vi "Blowout.vi"(10 "Blowout (ms)":u32=1500, 11 "Delay (ms)":u32) -> ()   [LabVIEW 2019]
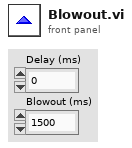
[diagram p1: front panel]
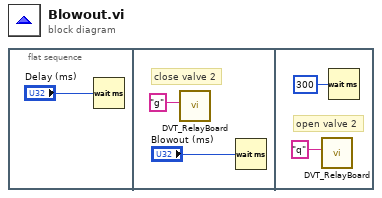
[diagram p0: block diagram]
diagram:
  n1 = flat-sequence {
    frame #0 {
      n2 = Wait (ms)(milliseconds to wait="Delay (ms)") -> ()  [unwired: 1 out]
    }
    frame #1 {
      # "close valve 2"
      n3 = call "DVT_RelayBoard.vi"("write buffer"="g") -> ()  [unwired: 3 in, 3 out]
      n4 = Wait (ms)(milliseconds to wait="Blowout (ms)") -> ()  [unwired: 1 out]
    }
    frame #2 {
      # "open valve 2"
      n5 = call "DVT_RelayBoard.vi"("write buffer"="q") -> ()  [unwired: 3 in, 3 out]
      n6 = Wait (ms)(milliseconds to wait=u32 300) -> ()  [unwired: 1 out]
    }
  }
